vi "Calibrate.vi"(8 "error in (no error)":errorcluster, 11 "Instrument in":refnum<class "Instrument Driver.lvclass">) -> (0 "error out":errorcluster, 1 "Success?":bool, 2 "Result":variant, 3 "Instrument out":refnum<class "Instrument Driver.lvclass">)   [LabVIEW 2020, in "Instrument Driver.lvlib" / "Instrument Driver.lvclass"]
doc: "Calibrate the instrument if supported. The calibration result is returned in a variant.\n\nThe default implementation does nothing."
uses:
  Instrument Driver.lvclass
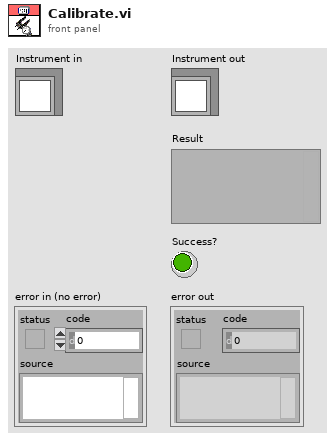
[diagram p1: front panel]
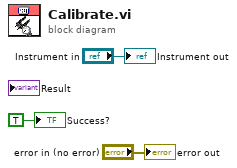
[diagram p0: block diagram]
diagram:
  "error out" <- "error in (no error)"
  "Instrument out" <- "Instrument in"
  "Success?" <- TRUE ("Success?")
